vi "Teleop.vi"(10 "Match Info":T1={"Autonomous Elapsed Seconds"=0.0, "TeleOp Elapsed Seconds"=0.0, "Disabled Elapsed Seconds"=0.0, "Visited Autonomous"=FALSE, "Visited TeleOp"=FALSE, "Visited Disabled"=FALSE, "Autonomous Settings"={"Autonomous Style"=enum."Independent", "VI Refnum"=refnum}}, 11 "Call Context":T2) -> ()   [LabVIEW 2013]
doc: "This VI is called for each TeleOp packet received from the DS where the robot is not disabled. It is often used to read from the joysticks and update I/O or to update setpoints for timed control loops. It should complete and return within 20 milliseconds or it may miss DS packets."
uses:
  Robot Global Data.vi
  <vilib>/Rock Robotics/WPI/Solenoid/WPI_SolenoidValue.ctl
  POT.vi
  Voltage.vi
  <vilib>/Rock Robotics/WPI/Solenoid/WPI_SolenoidSetEnum.vi
  <vilib>/Rock Robotics/WPI/Solenoid/Deprecated/WPI_SolenoidGetBool.vi
  <vilib>/Rock Robotics/WPI/DriverStation/WPI_DriverStationMatch Info.ctl
  <vilib>/Rock Robotics/WPI/DriverStation/WPI_DriverStationDerivedRobotMode.ctl
panel:
  out "Voltage":dbl
  out "POT Value  2":dbl
  out "POT Value 3":dbl
  out "POT Value":dbl
  out "Numeric 1":dbl(slide) scale=0.0..100.0
  out "Boolean 2":bool
  out "Boolean 1":bool
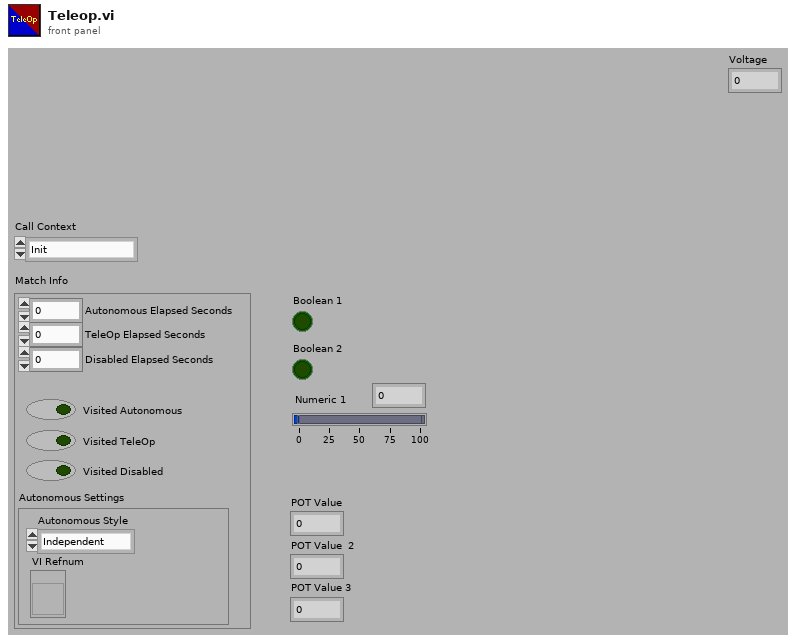
[diagram p1: front panel]
types:
  T1 = typedef "WPI_DriverStationMatch Info.ctl" = cluster{"Autonomous Elapsed Seconds":dbl, "TeleOp Elapsed Seconds":dbl, "Disabled Elapsed Seconds":dbl, "Visited Autonomous":bool, "Visited TeleOp":bool, "Visited Disabled":bool, "Autonomous Settings":cluster{"Autonomous Style":enum16{"Iterative", "Independent"}, "VI Refnum":refnum<vi>}}
  T2 = typedef "WPI_DriverStationDerivedRobotMode.ctl" = enum16{"Init", "Execute", "Stop"}
  T3 = typedef "WPI_JoystickDevRef.ctl" = cluster{"Device":T4}
  T4 = typedef "WPI_JoystickDeviceEnum.ctl" = enum16{"USB 1", "USB 2", "USB 3", "USB 4", "Kinect 1", "Kinect 2"}
  T5 = typedef "WPI_JoystickButtonState.ctl" = cluster{"Button 1":bool, "Button 2":bool, "Button 3":bool, "Button 4":bool, "Button 5":bool, "Button 6":bool, "Button 7":bool, "Button 8":bool, "Button 9":bool, "Button 10":bool, "Button 11":bool, "Button 12":bool}
  T6 = typedef "WPI_SolenoidDevRef.ctl" = cluster{"DevStatus":errorcluster, "Solenoid Module":T7, "Forward Solenoid Channel":T8, "Reverse Solenoid Channel":T8}
  T7 = typedef "FPGA_TypedefSolenoidModule.ctl" = enum16{"Solenoid Module 1", "Solenoid Module 2"}
  T8 = typedef "WPI_SolenoidChannel.ctl" = enum8{"Solenoid 1", "Solenoid 2", "Solenoid 3", "Solenoid 4", "Solenoid 5", "Solenoid 6", "Solenoid 7", "Solenoid 8", "Invalid"}
  T9 = typedef "WPI_SolenoidValue.ctl" = enum16{"Off", "On", "Forward", "Reverse"}
  T10 = typedef "WPI_MotorControlDeviceRef.ctl" = cluster{"DeviceStatus":errorcluster, "Type":enum16{"PWM", "CAN"}, "PWM":cluster{"Digital Module":T11, "PWM Channel":T12, "DeadBand":T13}, "CAN":cluster{"Device Number":u8, "Control Mode":T14, "Semaphore":T15, "Max Vout":dbl}, "Invert":bool, "TransformRef":T16, "InvTransformRef":T16}
  T11 = typedef "FPGA_TypedefDigitalModule.ctl" = enum16{"Digital Module 1", "Digital Module 2"}
  T12 = typedef "FPGA_DIOPWMChannel.ctl" = enum8{"PWM 1", "PWM 2", "PWM 3", "PWM 4", "PWM 5", "PWM 6", "PWM 7", "PWM 8", "PWM 9", "PWM 10", "Invalid"}
  T13 = typedef "WPI_PWMDeadband.ctl" = cluster{"Name":string, "maxPositivePwm":i32, "minPositivePwm":i32, "centerPwm":i32, "maxNegativePwm":i32, "minNegativePwm":i32, "angularRange":u16}
  T14 = typedef "WPI_CANJaguar_ControlMode.ctl" = enum8{"Percent VBus", "Current", "Speed", "Position", "Voltage"}
  T15 = typedef "Semaphore RefNum" = refnum<k1>
  T16 = typedef "WPI_PWMTransform_ConPane.ctl" = refnum<vi>
  T17 = typedef "WPI_RobotDriveDevRef.ctl" = cluster{"DevStatus":errorcluster, "Motors[]":T10[], "Square Inputs":bool, "Max Output":dbl, "Isochronous":bool}
  T18 = cluster{"axis 1 (x)":dbl, "axis 2 (y)":dbl, "axis 3 (throttle)":dbl, "axis 4":dbl, "axis 5":dbl, "axis 6":dbl}
  T19 = typedef "WPI_RelayDevRef.ctl" = cluster{"DevStatus":errorcluster, "Relay Channel":T20, "Digital Module":T11, "Relay Direction":T21}
  T20 = typedef "FPGA_DIORelayChannel.ctl" = enum8{"Relay 1", "Relay 2", "Relay 3", "Relay 4", "Relay 5", "Relay 6", "Relay 7", "Relay 8", "Invalid"}
  T21 = typedef "WPI_RelayDirection.ctl" = enum16{"Both directions", "Forward only", "Reverse only"}
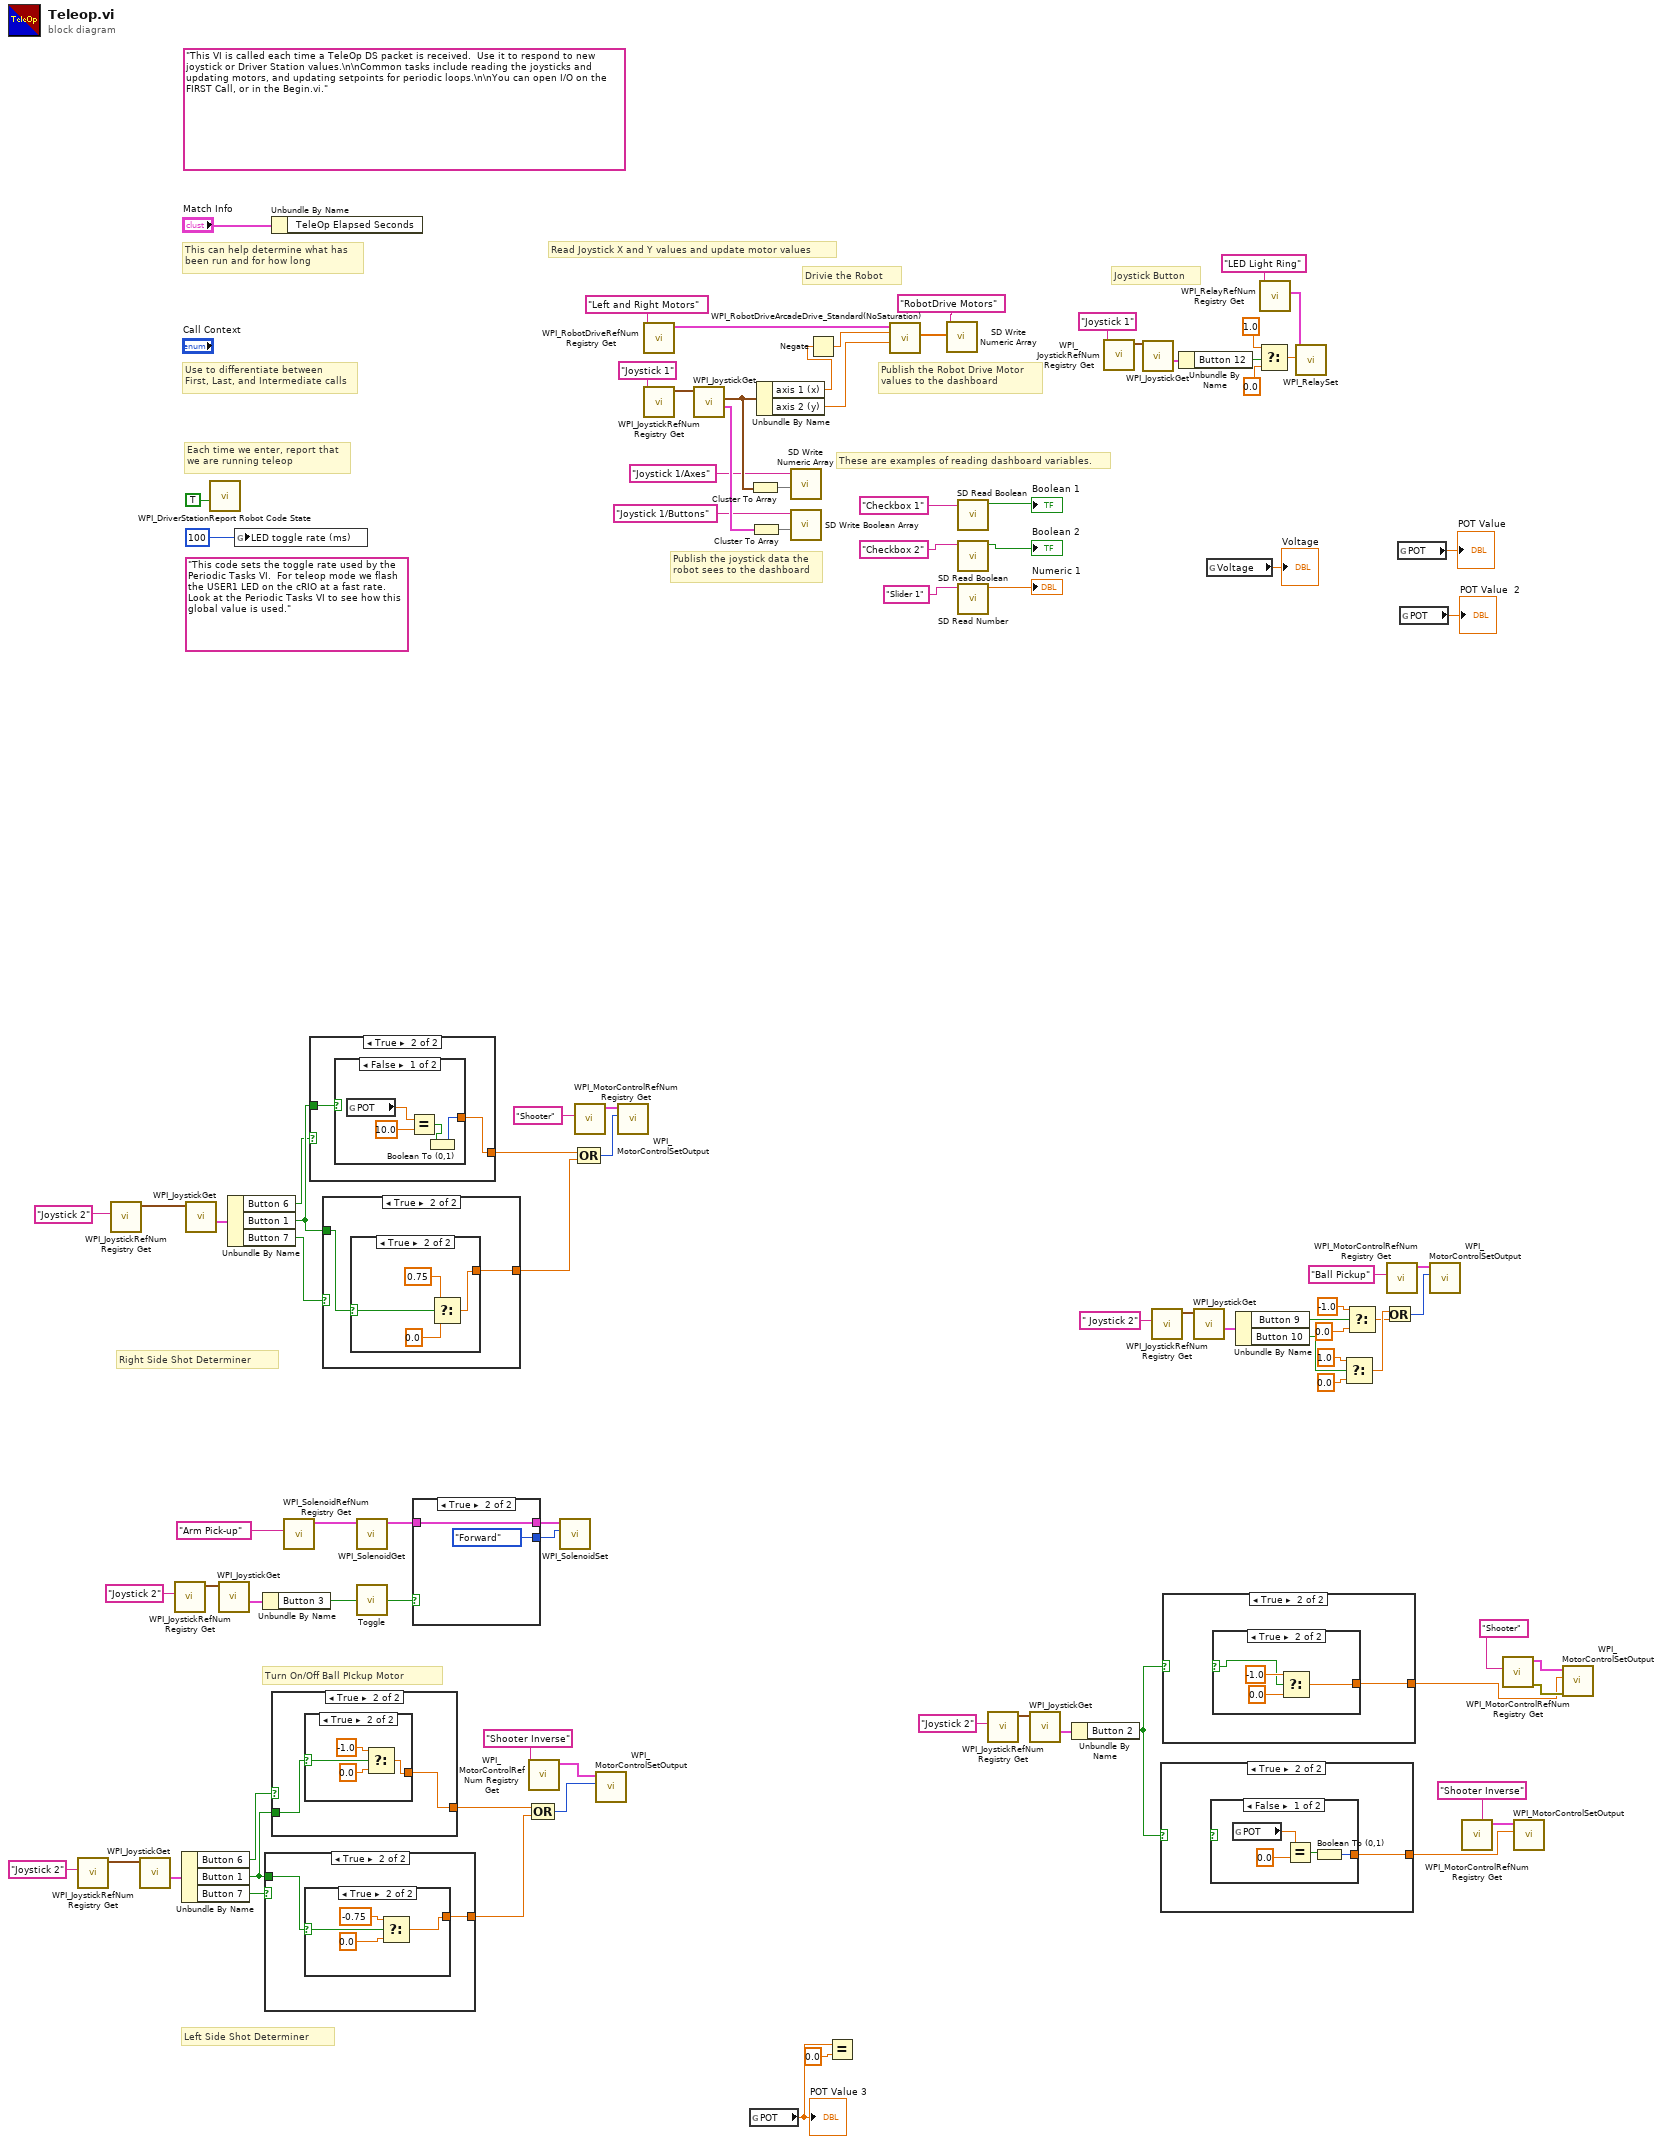
[diagram p0: block diagram]
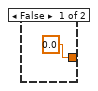
[diagram p2: hidden frame]
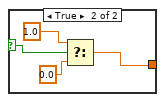
[diagram p3: hidden frame]
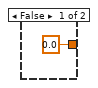
[diagram p4: hidden frame]
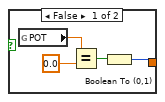
[diagram p5: hidden frame]
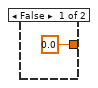
[diagram p6: hidden frame]
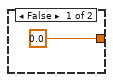
[diagram p7: hidden frame]
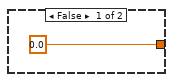
[diagram p8: hidden frame]
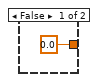
[diagram p9: hidden frame]
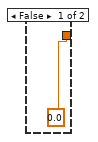
[diagram p10: hidden frame]
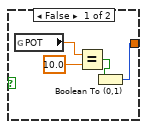
[diagram p11: hidden frame]
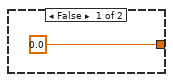
[diagram p12: hidden frame]
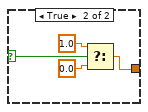
[diagram p13: hidden frame]
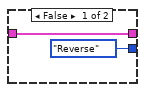
[diagram p14: hidden frame]
diagram:
  (unwired) "This code sets the toggle rate used by the Periodic Tasks VI.  For teleop mode we flash the USER1 LED on the cRIO at a fast rate.  Look at the Periodic Tasks VI to see how this global value is used."
  (unwired) "This VI is called each time a TeleOp DS packet is received.  Use it to respond to new joystick or Driver Station values.\n\nCommon tasks include reading the joysticks and updating motors, and updating setpoints for periodic loops.\n\nYou can open I/O on the FIRST Call, or in the Begin.vi."
  # "Left Side Shot Determiner"
  # "Right Side Shot Determiner"
  # "Turn On/Off Ball PIckup Motor"
  # "Joystick Button"
  # "Drivie the Robot"
  # "These are examples of reading dashboard variables."
  # "Publish the Robot Drive Motor\nvalues to the dashboard"
  # "Publish the joystick data the\nrobot sees to the dashboard"
  # "Each time we enter, report that\nwe are running teleop"
  # "Use to differentiate between\nFirst, Last, and Intermediate calls"
  # "This can help determine what has\nbeen run and for how long"
  # "Read Joystick X and Y values and update motor values"
  n1 = call <vilib>:"WPI_JoystickRefNum Registry Get.vi"("refnum name"="Joystick 2") -> ("JoystickDevRef"=w10:T3)  [unwired: 9 in, 1 out]
  n2 = call <vilib>:"WPI_JoystickRefNum Registry Get.vi"("refnum name"="Joystick 2") -> ("JoystickDevRef"=w9:T3)  [unwired: 9 in, 1 out]
  n3 = call <vilib>:"WPI_JoystickGet.vi"("JoystickDevRef"=w10) -> ("Buttons"=w11:T5)  [unwired: 4 in, 2 out]
  n4 = call <vilib>:"WPI_JoystickRefNum Registry Get.vi"("refnum name"="Joystick 2") -> ("JoystickDevRef"=w60:T3)  [unwired: 9 in, 1 out]
  n5 = Unbundle By Name(w11) -> ("Button 6"=w12:bool, "Button 1"=w14:bool, "Button 7"=w13:bool)
  n6 = call <vilib>:"WPI_JoystickGet.vi"("JoystickDevRef"=w9) -> ("Buttons"=w20:T5)  [unwired: 4 in, 2 out]
  n7 = call <vilib>:"WPI_DriverStationReport Robot Code State.vi"("TeleOp"=TRUE ("Autonomous")) -> ()  [unwired: 10 in, 1 out]
  n8 = call <vilib>:"WPI_JoystickGet.vi"("JoystickDevRef"=w60) -> ("Buttons"=w59:T5)  [unwired: 4 in, 2 out]
  n9 = Unbundle By Name(w20) -> ("Button 6"=w21:bool, "Button 1"=w23:bool, "Button 7"=w22:bool)
  n10 = global write "Robot Global Data.vi" "LED toggle rate (ms)"(u32 100 ("LED ms toggle rate")) -> ()
  n11 = Unbundle By Name(w59) -> ("Button 3"=w56:bool)
  n12 = case shown="True" w13 {
    tunnel: w14 -> [_ w98]
    tunnel: [0.0 ("f") w97] -> w16
    frame False {
    }
    frame True {
      n13 = case shown="True" w98 {
        selector: w98 -> [_ w101]
        tunnel: [0.0 ("f") w100] -> w97
        frame False {
        }
        frame True {
          n14 = Select(t=-0.75, s=w101, f=0.0) -> (s? t:f=w100:dbl)
        }
      }
    }
  }
  n15 = Unbundle By Name("Match Info") -> ()  [unwired: 1 out]
  n16 = case shown="True" w12 {
    tunnel: w14 -> [_ w106]
    tunnel: [0.0 ("f") w105] -> w15
    frame False {
    }
    frame True {
      n17 = case shown="True" w106 {
        selector: w106 -> [_ w109]
        tunnel: [0.0 ("f") w108] -> w105
        frame False {
        }
        frame True {
          n18 = Select(t=-1.0, s=w109, f=0.0) -> (s? t:f=w108:dbl)
        }
      }
    }
  }
  n19 = call <vilib>:"WPI_SolenoidRefNum Registry Get.vi"("refnum name"="Arm Pick-up") -> ("SolenoidDevRef"=w43:T6)  [unwired: 9 in, 1 out]
  n20 = case shown="True" w21 {
    tunnel: w23 -> [_ w114]
    tunnel: [0.0 ("f") w113] -> w24
    frame False {
    }
    frame True {
      n21 = case shown="False" w114 {
        selector: w114 -> [_ w120]
        tunnel: [w115 w119] -> w113
        frame False {
          n22 = global read "POT.vi" "POT"() -> (w118:dbl)
          n23 = Equal?(x=w118, y=10.0) -> (x = y?=w116:bool)
          n24 = Boolean To (0,1)(Boolean=w116) -> (0, 1=w115:i16)
        }
        frame True {
          n25 = Select(t=1.0, s=w120, f=0.0) -> (s? t:f=w119:dbl)
        }
      }
    }
  }
  n26 = case shown="True" w22 {
    tunnel: w23 -> [_ w125]
    tunnel: [0.0 ("f") w124] -> w25
    frame False {
    }
    frame True {
      n27 = case shown="True" w125 {
        selector: w125 -> [_ w131]
        tunnel: [w126 w130] -> w124
        frame False {
          n28 = global read "POT.vi" "POT"() -> (w127:dbl)
          n29 = Equal?(x=w127, y=10.0) -> (x = y?=w129:bool)
          n30 = Boolean To (0,1)(Boolean=w129) -> (0, 1=w126:i16)
        }
        frame True {
          n31 = Select(t=0.75, s=w131, f=0.0) -> (s? t:f=w130:dbl)
        }
      }
    }
  }
  n32 = call-poly <vilib>:"WPI_SolenoidGet.vi"("SolenoidDevRef"=w43) -> ("SolenoidDevRef"=w41:T6)  [unwired: 8 in, 2 out]
  n33 = call "Toggle.vi"("Input"=w56) -> ("Toggled Output"=w42:bool)
  n34 = case shown="True" w42 {
    tunnel: w41 -> [w135 w137]
    tunnel: [w135 w137] -> w40
    tunnel: [WPI_SolenoidValue."Reverse" ("Value") WPI_SolenoidValue."Forward" ("Value")] -> w39
    frame False {
    }
    frame True {
    }
  }
  n35 = call <vilib>:"WPI_MotorControlRefNum Registry Get.vi"("refnum name"="Shooter Inverse") -> ("MotorControlDevRef"=w19:T10)  [unwired: 9 in, 1 out]
  n36 = Compound Arithmetic op=OR(w15, w16) -> (w17:i32)
  n37 = call-poly <vilib>:"WPI_SolenoidSet.vi"("Value"=w39, "SolenoidDevRef"=w40) -> ()  [unwired: 8 in, 2 out]
  n38 = call <vilib>:"WPI_MotorControlRefNum Registry Get.vi"("refnum name"="Shooter") -> ("MotorControlDevRef"=w28:T10)  [unwired: 9 in, 1 out]
  n39 = Compound Arithmetic op=OR(w24, w25) -> (w26:i32)
  n40 = call <vilib>:"WPI_MotorControlSetOutput.vi"("Output"=w17, "MotorControlDevRef"=w19) -> ()  [unwired: 7 in, 3 out]
  n41 = call <vilib>:"WPI_MotorControlSetOutput.vi"("Output"=w26, "MotorControlDevRef"=w28) -> ()  [unwired: 7 in, 3 out]
  n42 = call <vilib>:"WPI_RobotDriveRefNum Registry Get.vi"("refnum name"="Left and Right Motors") -> ("RobotDriveDevRef"=w93:T17)  [unwired: 1 in, 9 out]
  n43 = call <vilib>:"WPI_JoystickRefNum Registry Get.vi"("refnum name"="Joystick 1") -> ("JoystickDevRef"=w90:T3)  [unwired: 1 in, 9 out]
  n44 = call <vilib>:"WPI_JoystickGet.vi"("JoystickDevRef"=w90) -> ("Buttons"=w87:T5, "Axes"=w84:T18)  [unwired: 1 in, 4 out]
  n45 = Cluster To Array(cluster=w84) -> (array=w83:dbl[])
  n46 = global read "POT.vi" "POT"() -> (w33:dbl)
  "POT Value 3" <- w33
  n47 = Cluster To Array(cluster=w87) -> (array=w86:bool[])
  n48 = Unbundle By Name(w84) -> ("axis 1 (x)"=w58:dbl, "axis 2 (y)"=w92:dbl)
  n49 = call <vilib>:"SD Write Numeric Array.vi"("Numeric Array"=w83, "Name"="Joystick 1/Axes") -> ()  [unwired: 8 in, 2 out]
  n50 = call <vilib>:"SD Write Boolean Array.vi"("Boolean Array"=w86, "Name"="Joystick 1/Buttons") -> ()  [unwired: 8 in, 2 out]
  n51 = Negate(x=w58) -> (-x=w57:dbl)
  n52 = Equal?(x=w33, y=0.0) -> ()  [unwired: 1 out]
  n53 = call <vilib>:"WPI_RobotDriveArcadeDrive_Standard(NoSaturation).vi"("Y axis value"=w92, "X axis value"=w57, "RobotDriveDevRef"=w93) -> ("Motor Values"=w80:dbl[])  [unwired: 1 in, 7 out]
  n54 = call <vilib>:"SD Write Numeric Array.vi"("Numeric Array"=w80, "Name"="RobotDrive Motors") -> ()  [unwired: 8 in, 2 out]
  n55 = call <vilib>:"SD Read Boolean.vi"("Name"="Checkbox 1" ("refnum name")) -> ("Boolean"=→"Boolean 1":bool)  [unwired: 8 in, 2 out]
  n56 = call <vilib>:"SD Read Boolean.vi"("Name"="Checkbox 2" ("refnum name")) -> ("Boolean"=→"Boolean 2":bool)  [unwired: 8 in, 2 out]
  n57 = call <vilib>:"SD Read Number.vi"("Name"="Slider 1" ("refnum name")) -> ("Numeric"=→"Numeric 1":dbl)  [unwired: 8 in, 2 out]
  n58 = call <vilib>:"WPI_JoystickRefNum Registry Get.vi"("refnum name"="Joystick 2") -> ("JoystickDevRef"=w35:T3)  [unwired: 9 in, 1 out]
  n59 = call <vilib>:"WPI_JoystickGet.vi"("JoystickDevRef"=w35) -> ("Buttons"=w34:T5)  [unwired: 4 in, 2 out]
  n60 = Unbundle By Name(w34) -> ("Button 2"=w6:bool)
  n61 = call <vilib>:"WPI_JoystickRefNum Registry Get.vi"("refnum name"="Joystick 1") -> ("JoystickDevRef"=w69:T3)  [unwired: 9 in, 1 out]
  n62 = call <vilib>:"WPI_JoystickGet.vi"("JoystickDevRef"=w69) -> ("Buttons"=w68:T5)  [unwired: 4 in, 2 out]
  n63 = call <vilib>:"WPI_JoystickRefNum Registry Get.vi"("refnum name"=" Joystick 2") -> ("JoystickDevRef"=w49:T3)  [unwired: 9 in, 1 out]
  n64 = case shown="True" w6 {
    tunnel: [0.0 ("f") w139] -> w2
    frame False {
    }
    frame True {
      n65 = case shown="False" {
        selector: _ -> [_ w147]
        tunnel: [w140 w144] -> w139
        frame False {
          n66 = global read "POT.vi" "POT"() -> (w143:dbl)
          n67 = Equal?(x=w143, y=0.0) -> (x = y?=w141:bool)
          n68 = Boolean To (0,1)(Boolean=w141) -> (0, 1=w140:i16)
        }
        frame True {
          n69 = Select(t=1.0, s=w147, f=0.0) -> (s? t:f=w144:dbl)
        }
      }
    }
  }
  n70 = case shown="True" w6 {
    tunnel: [0.0 ("f") w149] -> w1
    frame False {
    }
    frame True {
      n71 = case shown="True" {
        selector: _ -> [_ w155]
        tunnel: [w150 w154] -> w149
        frame False {
          n72 = global read "POT.vi" "POT"() -> (w152:dbl)
          n73 = Equal?(x=w152, y=0.0) -> (x = y?=w151:bool)
          n74 = Boolean To (0,1)(Boolean=w151) -> (0, 1=w150:i16)
        }
        frame True {
          n75 = Select(t=-1.0, s=w155, f=0.0) -> (s? t:f=w154:dbl)
        }
      }
    }
  }
  n76 = Unbundle By Name(w68) -> ("Button 12"=w67:bool)
  n77 = call <vilib>:"WPI_JoystickGet.vi"("JoystickDevRef"=w49) -> ("Buttons"=w50:T5)  [unwired: 4 in, 2 out]
  n78 = global read "Voltage.vi" "Voltage"() -> (→"Voltage":dbl)
  n79 = Unbundle By Name(w50) -> ("Button 9"=w51:bool, "Button 10"=w47:bool)
  n80 = Select(t=1.0, s=w67, f=0.0) -> (s? t:f=w66:dbl)
  n81 = call <vilib>:"WPI_RelayRefNum Registry Get.vi"("refnum name"="LED Light Ring") -> ("RelayDevRef"=w73:T19)  [unwired: 9 in, 1 out]
  n82 = call <vilib>:"WPI_RelaySet.vi"("RelayValue"=w66, "RelayDevRef"=w73) -> ()  [unwired: 8 in, 2 out]
  n83 = Select(t=1.0, s=w47, f=0.0) -> (s? t:f=w46:dbl)
  n84 = Select(t=-1.0, s=w51, f=0.0) -> (s? t:f=w45:dbl)
  n85 = Or(x=w46, y=w45) -> (x .or. y?=w44:i32)
  n86 = call <vilib>:"WPI_MotorControlRefNum Registry Get.vi"("refnum name"="Ball Pickup") -> ("MotorControlDevRef"=w63:T10)  [unwired: 9 in, 1 out]
  n87 = global read "POT.vi" "POT"() -> (→"POT Value":dbl)
  n88 = global read "POT.vi" "POT"() -> (→"POT Value  2":dbl)
  n89 = call <vilib>:"WPI_MotorControlSetOutput.vi"("Output"=w44, "MotorControlDevRef"=w63) -> ()  [unwired: 7 in, 3 out]
  n90 = call <vilib>:"WPI_MotorControlRefNum Registry Get.vi"("refnum name"="Shooter Inverse") -> ("MotorControlDevRef"=w3:T10)  [unwired: 9 in, 1 out]
  n91 = call <vilib>:"WPI_MotorControlRefNum Registry Get.vi"("refnum name"="Shooter") -> ("error out"=w5:errorcluster, "MotorControlDevRef"=w4:T10)  [unwired: 9 in]
  n92 = call <vilib>:"WPI_MotorControlSetOutput.vi"("Output"=w2, "MotorControlDevRef"=w3) -> ()  [unwired: 7 in, 3 out]
  n93 = call <vilib>:"WPI_MotorControlSetOutput.vi"("error in (no error)"=w5, "Output"=w1, "MotorControlDevRef"=w4) -> ()  [unwired: 6 in, 3 out]
